vi "AdditionalDescription.vi"(8 "error in":errorcluster, 11 "Vi":path) -> (0 "error out":errorcluster, 3 "Additonal Description":string)   [LabVIEW 2020]
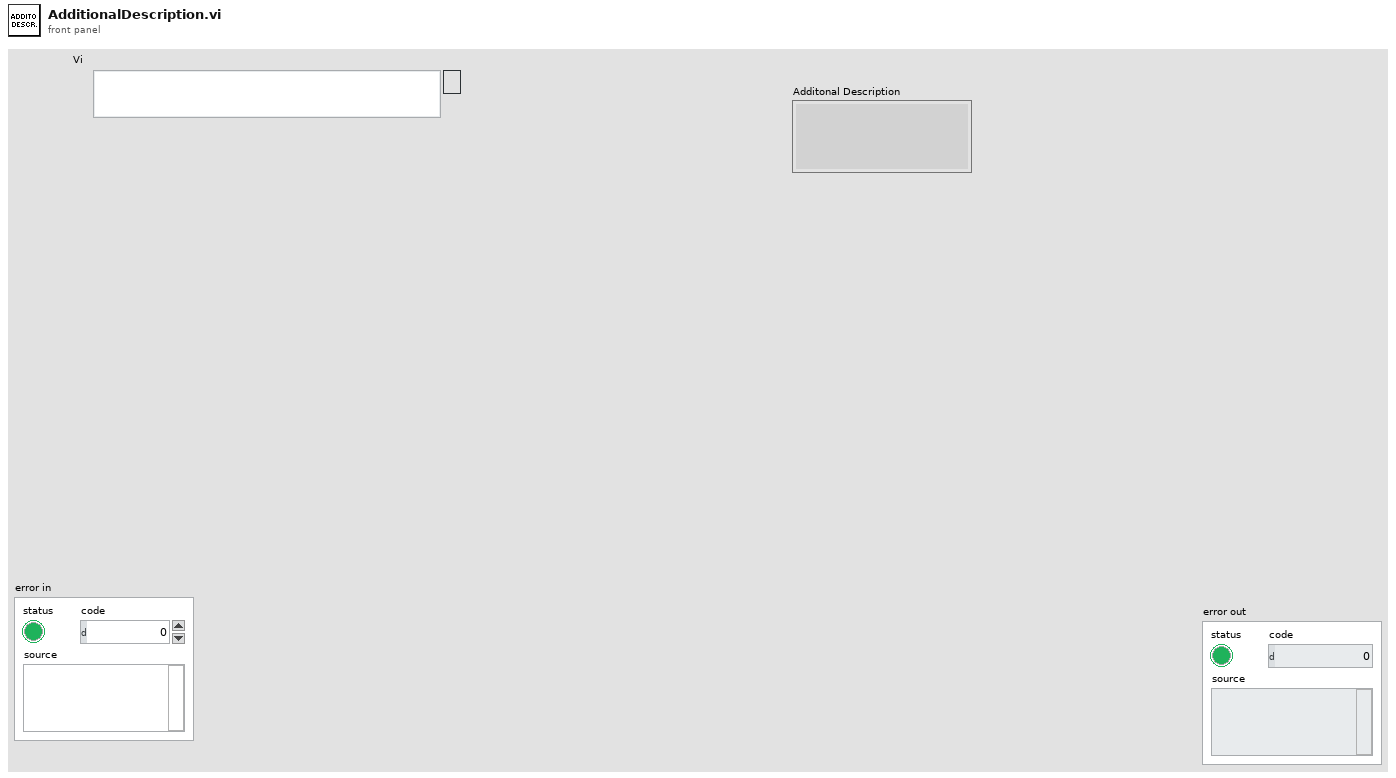
[diagram p1: front panel]
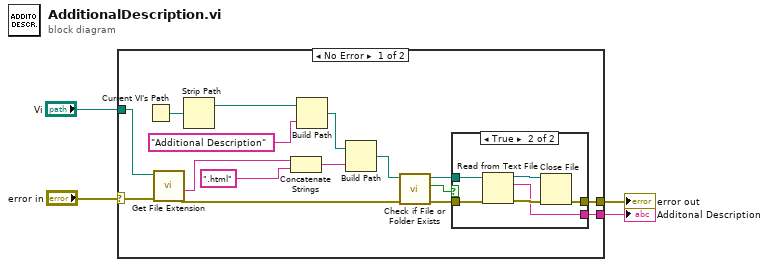
[diagram p0: block diagram]
diagram:
  n1 = case shown="No Error" "error in" {
    selector: "error in" -> [w15 w28]
    tunnel: [w20 w28] -> w3
    tunnel: "Vi" -> [w14 _]
    tunnel: [w19 _] -> w1
    frame No Error {
      n2 = Current VI's Path() -> (path=w18:path)
      n3 = call <vilib>:"Get File Extension.vi"("error in (no error)"=w15, "file"=w14) -> ("error out"=w9:errorcluster, "filename without extension"=w12:string)  [unwired: 5 in, 3 out]
      n4 = Strip Path(path=w18) -> (stripped path=w17:path)  [unwired: 1 out]
      n5 = Concatenate Strings(w12, ".html") -> (w11:string)
      n6 = Build Path(base path=w17, name or relative path="Additional Description") -> (appended path=w13:path)
      n7 = Build Path(base path=w13, name or relative path=w11) -> (appended path=w8:path)
      n8 = call <vilib>:"Check if File or Folder Exists.vi"("error in (no error)"=w9, "path"=w8) -> ("error out"=w7:errorcluster, "file or folder exists?"=w5:bool, "dup path"=w6:path)  [unwired: 7 in]
      n9 = case shown="True" w5 {
        tunnel: [w21 w25] -> w20
        tunnel: [_ w24] -> w19
        tunnel: w7 -> [w21 w23]
        tunnel: w6 -> [_ w22]
        frame False {
          # "no file"
        }
        frame True {
          n10 = Read from Text File(file (use dialog)=w22, error in=w23) -> (refnum out=w26:refnum<file>, text=w24:string, error out=w27:errorcluster)  [unwired: 2 in, 1 out]
          n11 = Close File(refnum=w26, error in=w27) -> (error out=w25:errorcluster)  [unwired: 1 out]
        }
      }
    }
    frame Error {
    }
  }
  "error out" <- w3
  "Additonal Description" <- w1
